vi "Read User-Defined States.vi"(8 "error in (no error)":errorcluster, 11 "CSM-Helper in":refnum<class "CSM-Helper.lvclass">) -> (0 "error out":errorcluster, 2 "Array":string[](array[string]), 3 "CSM-Helper out":refnum<class "CSM-Helper.lvclass">)   [LabVIEW 2020, in "CSM-Helper.lvclass"]
uses:
  CSM-Helper.lvclass
  CSM-Helper.lvclass/CSM-Helper.ctl
  <userlib>/_NEVSTOP/Communicable State Machine(CSM)/Communicable State Machine.lvlib
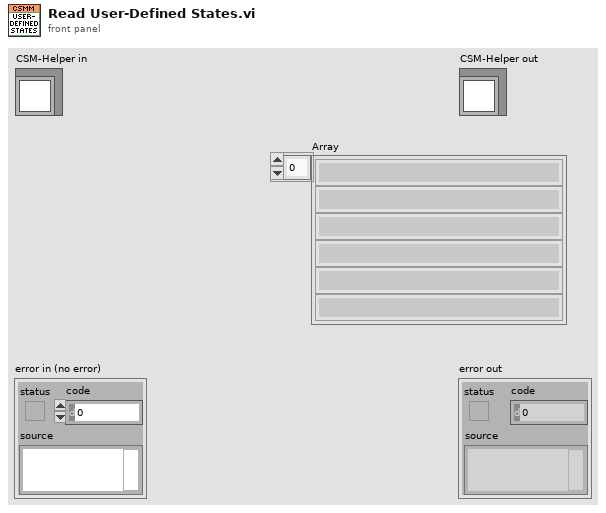
[diagram p1: front panel]
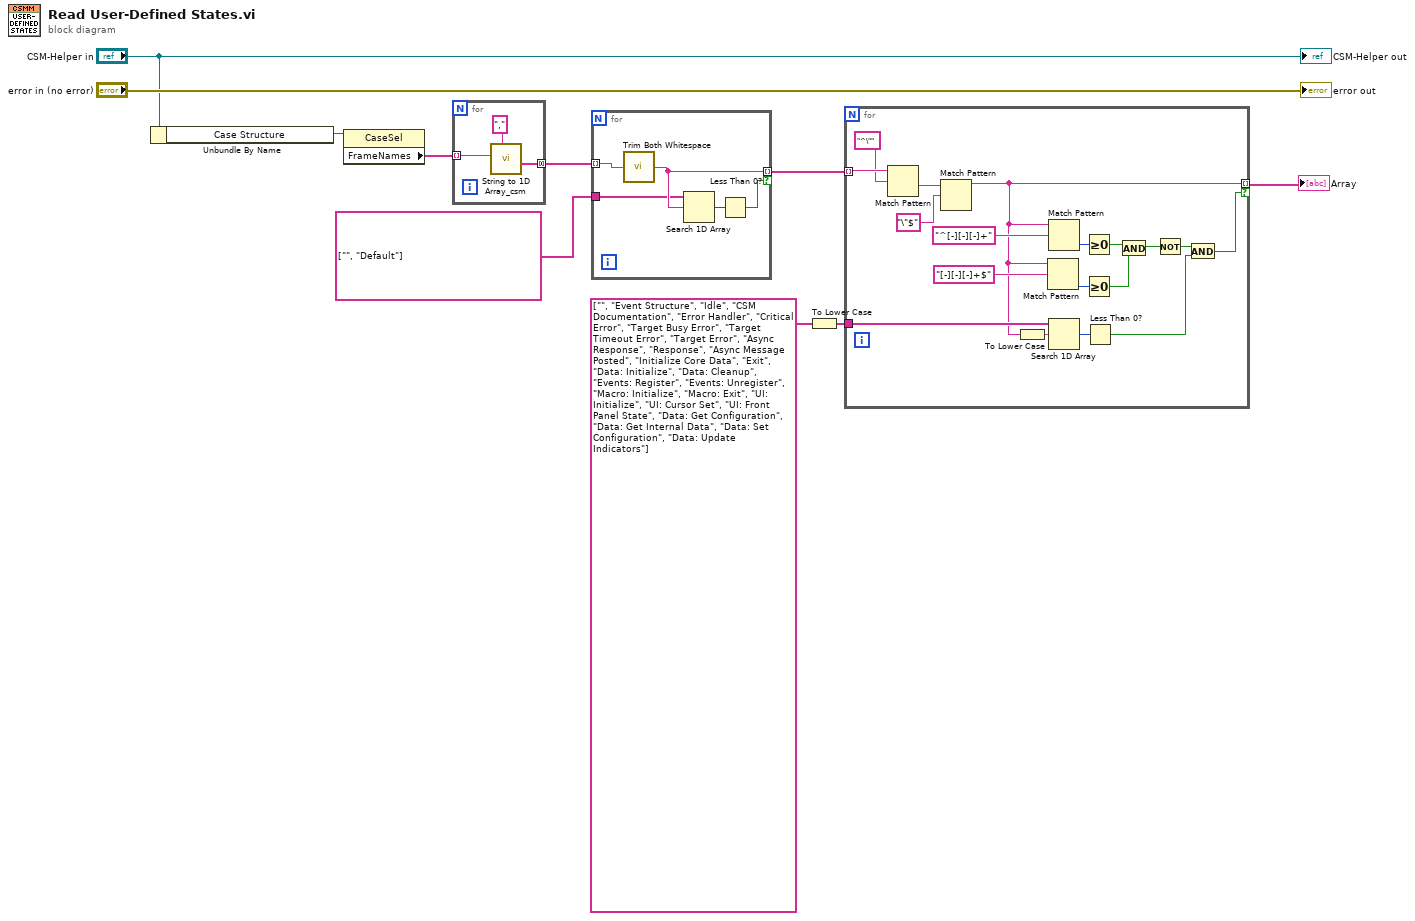
[diagram p0: block diagram]
diagram:
  n1 = Unbundle By Name("CSM-Helper in") -> ("Case Structure"=w8:refnum<vi>)
  n2 = property on="Property Node" class="CaseSel"(reference=w8) -> ("FrameNames"=w7:string[])  [unwired: 1 in, 2 out]
  n3 = for {
    tunnel: w7 -> [w13] mode=indexing
    tunnel: [w11] -> w6 mode=concatenating
    n4 = call <userlib>:"String to 1D Array_csm.vi"("delimiter (Tab)"=",", "string"=w13) -> ("Array of Strings"=w11:string[])  [unwired: 9 in]
  }
  n5 = for {
    tunnel: w6 -> [w18] mode=indexing
    tunnel: [w16] -> w4 mode=indexing if=w14
    tunnel: string[] ["", "Default"] ("items to filter") -> [w15]
    n6 = call <userlib>:"Trim Both Whitespace.vi"("string"=w18) -> ("trimmed string"=w16:string)  [unwired: 1 in]
    n7 = Search 1D Array(1D array=w15, element=w16) -> (index of element=w17:i32)  [unwired: 1 in]
    n8 = Less Than 0?(x=w17) -> (x < 0?=w14:bool)
  }
  n9 = To Lower Case(string=string[] ["", "Event Structure", "Idle", "CSM Documentation", "Error Handler", "Critical Error", "Target Busy Error", "Target Timeout Error", "Target Error", "Async Response", "Response", "Async Message Posted", "Initialize Core Data", "Exit", "Data: Initialize", "Data: Cleanup", "Events: Register", "Events: Unregister", "Macro: Initialize", "Macro: Exit", "UI: Initialize", "UI: Cursor Set", "UI: Front Panel State", "Data: Get Configuration", "Data: Get Internal Data", "Data: Set Configuration", "Data: Update Indicators"] ("items to filter")) -> (all lower case string=w1:string[])
  n10 = for {
    tunnel: w4 -> [w36] mode=indexing
    tunnel: [w22] -> w3 mode=indexing if=w20
    tunnel: w1 -> [w23]
    n11 = Match Pattern(string=w36, regular expression="^\"") -> (after substring=w34:string)  [unwired: 1 in, 3 out]
    n12 = Match Pattern(string=w34, regular expression="\"$") -> (before substring=w22:string)  [unwired: 1 in, 3 out]
    n13 = To Lower Case(string=w22) -> (all lower case string=w21:string)
    n14 = Match Pattern(string=w22, regular expression="[-][-][-]+$") -> (offset past match=w29:i32)  [unwired: 1 in, 3 out]
    n15 = Match Pattern(string=w22, regular expression="^[-][-][-]+") -> (offset past match=w30:i32)  [unwired: 1 in, 3 out]
    n16 = Search 1D Array(1D array=w23, element=w21) -> (index of element=w24:i32)  [unwired: 1 in]
    n17 = Greater Or Equal To 0?(x=w30) -> (x >= 0?=w28:bool)
    n18 = Greater Or Equal To 0?(x=w29) -> (x >= 0?=w27:bool)
    n19 = Less Than 0?(x=w24) -> (x < 0?=w19:bool)
    n20 = And(x=w28, y=w27) -> (x .and. y?=w26:bool)
    n21 = Not(x=w26) -> (.not. x?=w25:bool)
    n22 = And(x=w25, y=w19) -> (x .and. y?=w20:bool)
  }
  "Array" <- w3
  "error out" <- "error in (no error)"
  "CSM-Helper out" <- "CSM-Helper in"
